vi "StimulusParameters.vi"(0 "waveform?":bool, 4 "pulse duration":dbl, 5 "channel":u16, 6 "pulses per stimulus":u16=1, 7 "resource":string, 8 "ISI":dbl, 9 "stimulus duration":dbl, 10 "number":i32, 11 "delay":dbl) -> (2 "stimulus parameters":T1)   [LabVIEW 2014]
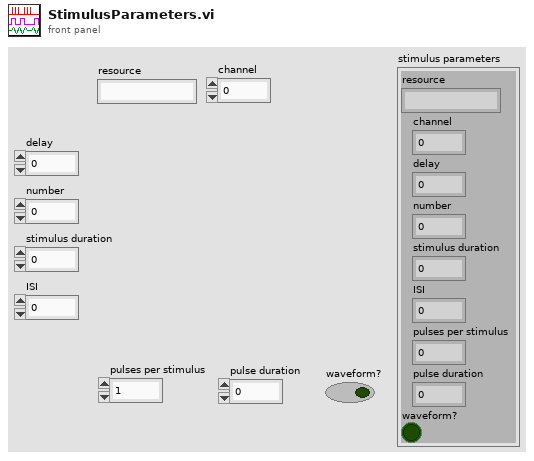
[diagram p1: front panel]
types:
  T1 = cluster{"resource":string, "channel":u16, "delay":dbl, "number":i32, "stimulus duration":dbl, "ISI":dbl, "pulses per stimulus":u16, "pulse duration":dbl, "waveform?":bool}
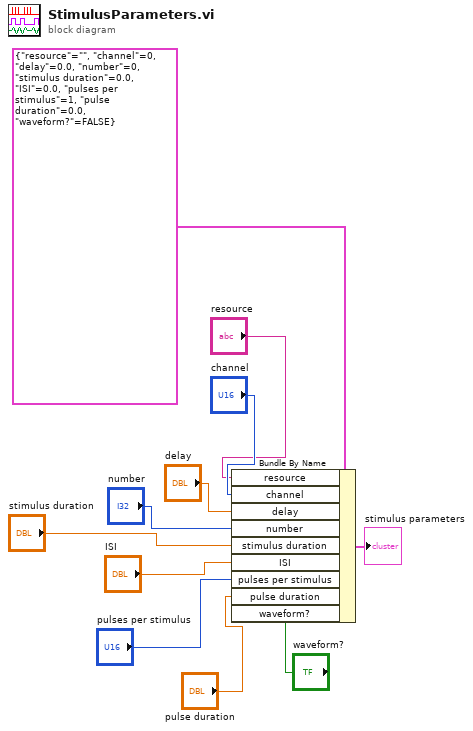
[diagram p0: block diagram]
diagram:
  n1 = Bundle By Name(cluster=T1 {"resource"="", "channel"=0, "delay"=0.0, "number"=0, "stimulus duration"=0.0, "ISI"=0.0, "pulses per stimulus"=1, "pulse duration"=0.0, "waveform?"=FALSE}, "resource"="resource", "channel"="channel", "delay"="delay", "number"="number", "stimulus duration"="stimulus duration", "ISI"="ISI", "pulses per stimulus"="pulses per stimulus", "pulse duration"="pulse duration", "waveform?"="waveform?") -> (→"stimulus parameters":T1)
